vi "Greater Equal.vi"(4 "Error":string, 5 "Output Image":T1={"Image ID"=0, "Channel ID"=-1}, 6 "Input Image 2":T1={"Image ID"=0, "Channel ID"=-1}, 7 "Input Image 1":T1={"Image ID"=0, "Channel ID"=-1}) -> (0 "Error":string, 1 "Output Image":T1={"Image ID"=0, "Channel ID"=-1}, 2 "Input Image 2":T1={"Image ID"=0, "Channel ID"=-1}, 3 "Input Image 1":T1={"Image ID"=0, "Channel ID"=-1})   [LabVIEW 2011, in "labvvis.lvlib"]
doc: "Adds each pixel from Input Image 1 with the corresponding pixel from Input Image 2. The result is written to Output Image. If the result is greater than 255, then the result is 255."
uses:
  <userlib>/labvvis/labvvis.lvlib
  <userlib>/labvvis/VVIS Image.ctl
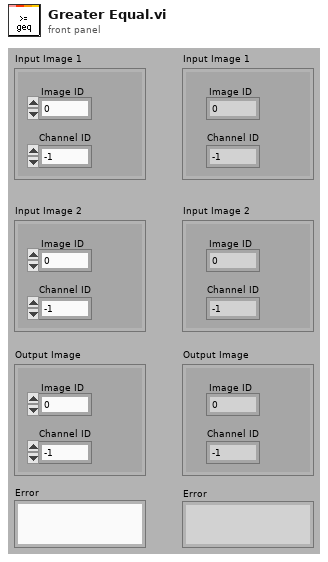
[diagram p1: front panel]
types:
  T1 = typedef "labvvis.lvlib/VVIS Image.ctl" = cluster{"Image ID":i16, "Channel ID":i16}
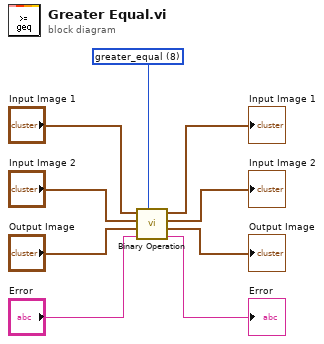
[diagram p0: block diagram]
diagram:
  w1 = u8 8 items=["plus_saturated", "minus_saturated", "multiplies", "divides", "modulus", "equal_to", "not_equal_to", "greater", "greater_equal", "less", "less_equal", "logical_and", "logical_or", "bitwise_and", "bitwise_or"] ("Function")
  n1 = call <userlib>:"Binary Operation.vi"("Function"=w1, "Error"="Error", "Output Image"="Output Image", "Input Image 2"="Input Image 2", "Input Image 1"="Input Image 1") -> ("Error"=→"Error":string, "Output Image"=→"Output Image":T1, "Input Image 2"=→"Input Image 2":T1, "Input Image 1"=→"Input Image 1":T1)
